vi "Replace 2D.vi"(7 "initialized 2D in":dbl[][](array[numeric]), 8 "error in":errorcluster, 9 "dimension size":i32=50, 10 "tc":u32, 11 "1D array":dbl[](array[numeric])) -> (0 "error out":errorcluster, 5 "initialized 2D out":dbl[][](array[numeric]))   [LabVIEW 2019, in "Zen Analytics.lvlib" / "Zen Analytics.lvclass"]
uses:
  Zen Analytics.lvclass
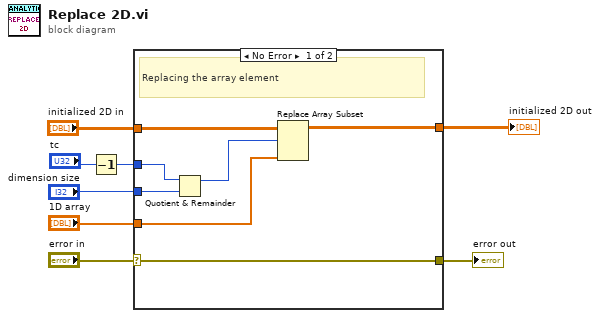
[diagram p0: block diagram]
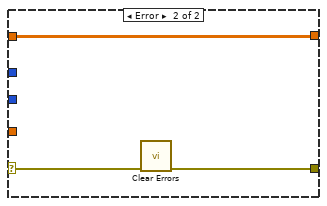
[diagram p2: hidden frame]
diagram:
  n1 = Decrement(x="tc") -> (x-1=w2:u32)
  n2 = case shown="No Error" "error in" {
    selector: "error in" -> [w15 w18]
    tunnel: [w15 w16] -> w1
    tunnel: "1D array" -> [w14 _]
    tunnel: w2 -> [w13 _]
    tunnel: "dimension size" -> [w12 _]
    tunnel: "initialized 2D in" -> [w11 w17]
    tunnel: [w9 w17] -> w3
    frame No Error {
      # "Replacing the array element"
      n3 = Quotient & Remainder(x=w13, y=w12) -> (x-y*floor(x/y)=w10:u32)  [unwired: 1 out]
      n4 = Replace Array Subset "Replace Array Subset"(array=w11, new element=w14, index (row)=w10) -> (w9:dbl[][])  [unwired: 1 in]
    }
    frame Error {
      n5 = call <vilib>:"Clear Errors.vi"("error in (no error)"=w18) -> ("error out"=w16:errorcluster)  [unwired: 5 in, 1 out]
    }
  }
  "error out" <- w1
  "initialized 2D out" <- w3
